vi "Process.vi"(0 "reference in":refnum<class "NI-DAQmx.lvclass">, 5 "error in (no error)":errorcluster) -> (14 "reference out":refnum<class "NI-DAQmx.lvclass">, 19 "error out":errorcluster)   [LabVIEW 2018, in "NI-DAQmx.lvclass"]
uses:
  NI-DAQmx.lvclass
  <vilib>/DAQmx/write.llb/DAQmx Write (Analog 1D DBL 1Chan NSamp).vi
  <vilib>/DAQmx/read.llb/DAQmx Read (Analog 1D Wfm NChan NSamp).vi
  <vilib>/Analysis/5stat.llb/RMS (DBL).vi
  <vilib>/DAQmx/miscellaneous.llb/DAQmx Fill In Error Info.vi
  <vilib>/measure/mascope.llb/Pulse Measurements 1 chan.vi
  <vilib>/measure/mascope.llb/Amplitude and Levels 1 chan.vi
  <resource>/objmgr/daqmx.rc
  <vilib>/measure/NI_MAPro.lvlib
  <vilib>/Analysis/NI_AALPro.lvlib
panel:
  out "Waveform Chart":dbl[][](graph)
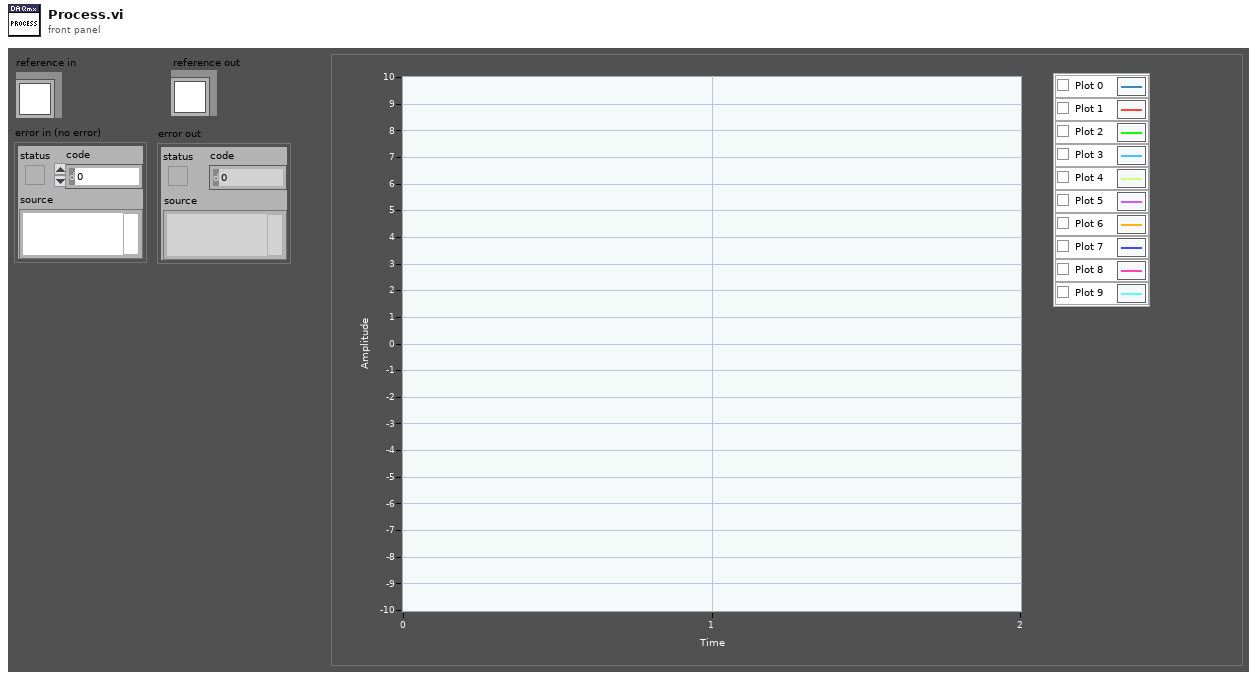
[diagram p1: front panel]
types:
  T1 = cluster{"Event":refnum<event-registration>, "Command":string, "Data":variant}
  T2 = typedef "NI-DAQmx.lvclass/ObjectAttributes.ctl" = cluster{"AI Task":refnum<k21>, "DO Task":refnum<k21>, "AO Task":refnum<k21>, "Latest Values":dbl[], "Signal List":T3[], "PWM Duty Cycle (%)":dbl, "PWM Amplitude (V)":dbl, "PWM Frequency (Hz)":dbl, "DO States":bool[]}
  T3 = typedef "IO Signal List.ctl" = enum16{"Timestamp", "PSU_FB_U_VDC", "PSU_FB_I_AMP", "PSU_FB_W_WATT", "PSU_CMD_U_VDC", "PSU_CMD_I_AMP", "PSU_CMD_OUTPUT", "LCR_PRIMARY", "LCR_SECONDARY", "UV_R_Ohm", "UW_R_Ohm", "VW_R_Ohm", "UV_L_H", "UW_L_H", "VW_L_H", "U_U_VDC", "V_U_VDC", "W_U_VDC", "U_I_AMP", "V_I_AMP", "W_I_AMP", "PWM_CMD_DC_%", "PWM_CMD_VDC", "PWM_CMD_Hz", "PWM_FB_DC_%", "PWM_FB_VDC", "PWM_FB_Hz", "DO_RELAY_U_LCR_A", "DO_RELAY_V_LCR_A", "DO_RELAY_V_LCR_B", "DO_RELAY_W_LCR_B", "DIFF_UV_UW_L_H", "DIFF_UV_VW_L_H", "DIFF_UW_VW_L_H", "DIFF_UV_UW_R_Ohm", "DIFF_UV_VW_R_Ohm", "DIFF_UW_VW_R_Ohm", "DIFF_UV_U_VDC", "DIFF_UW_U_VDC", "DIFF_VW_U_VDC"}
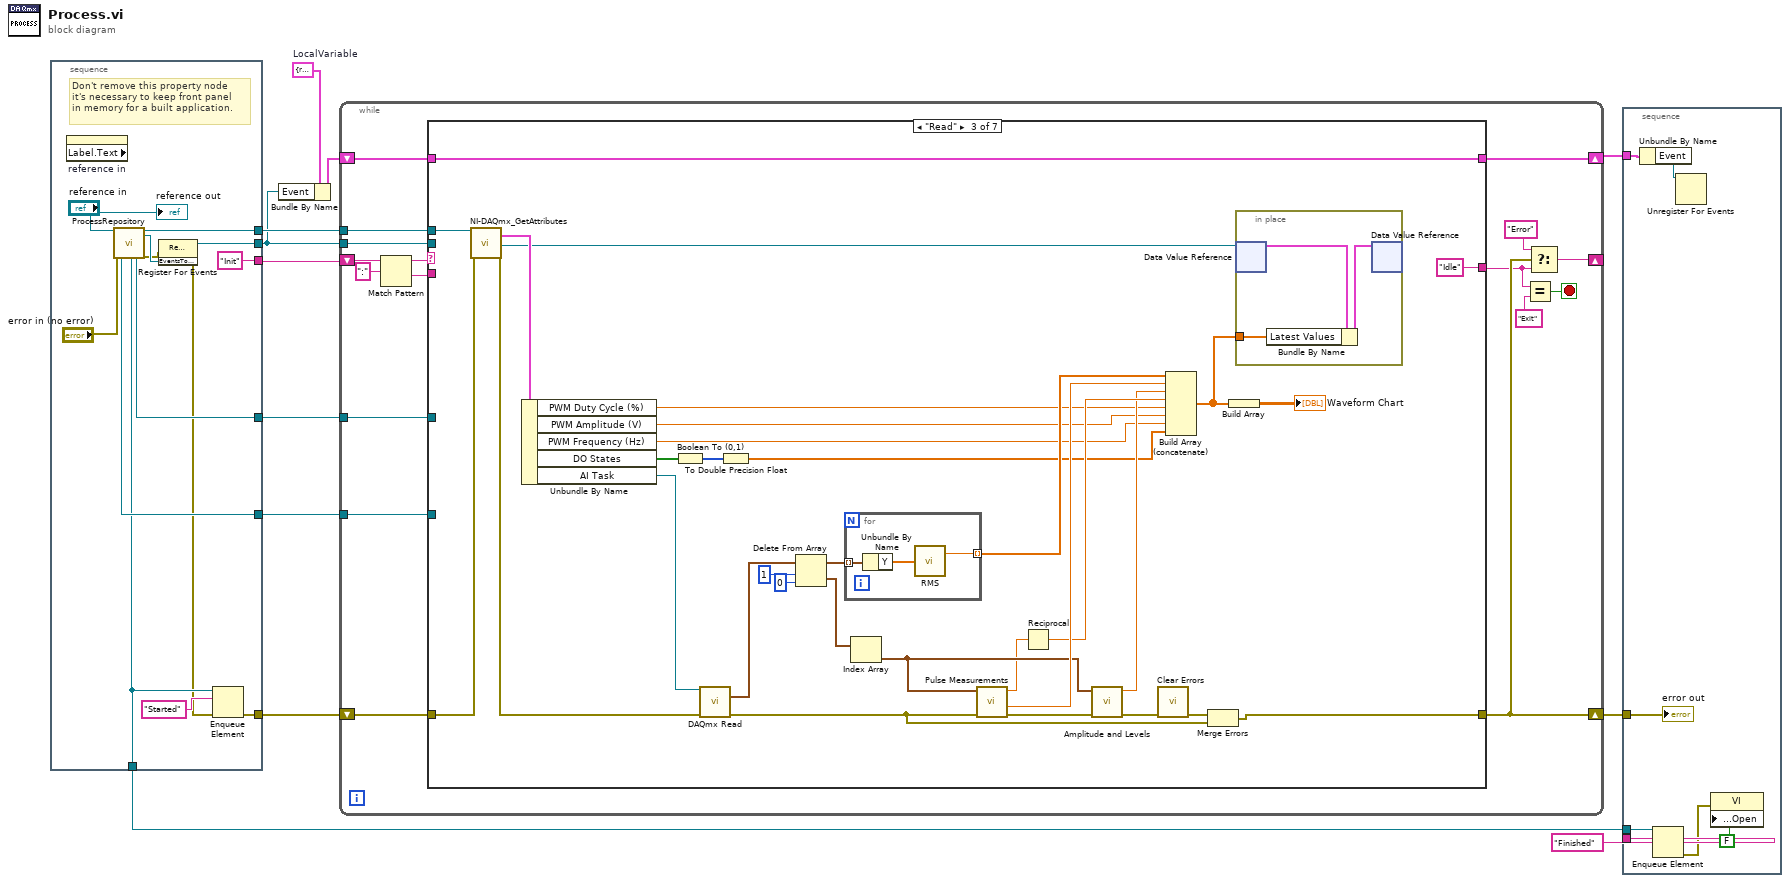
[diagram p0: block diagram]
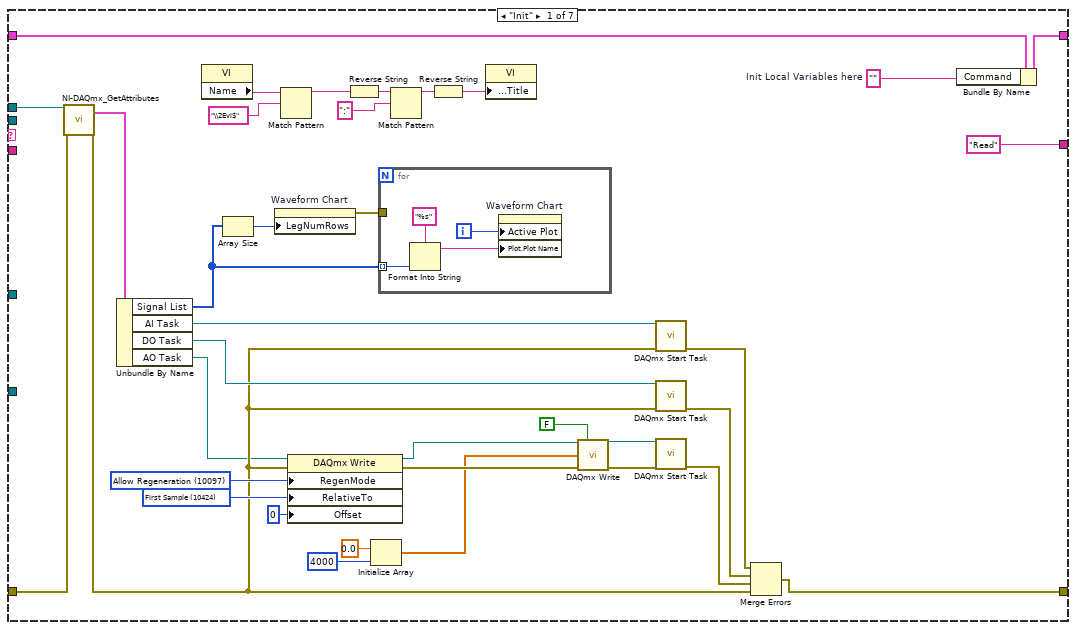
[diagram p2: hidden frame]
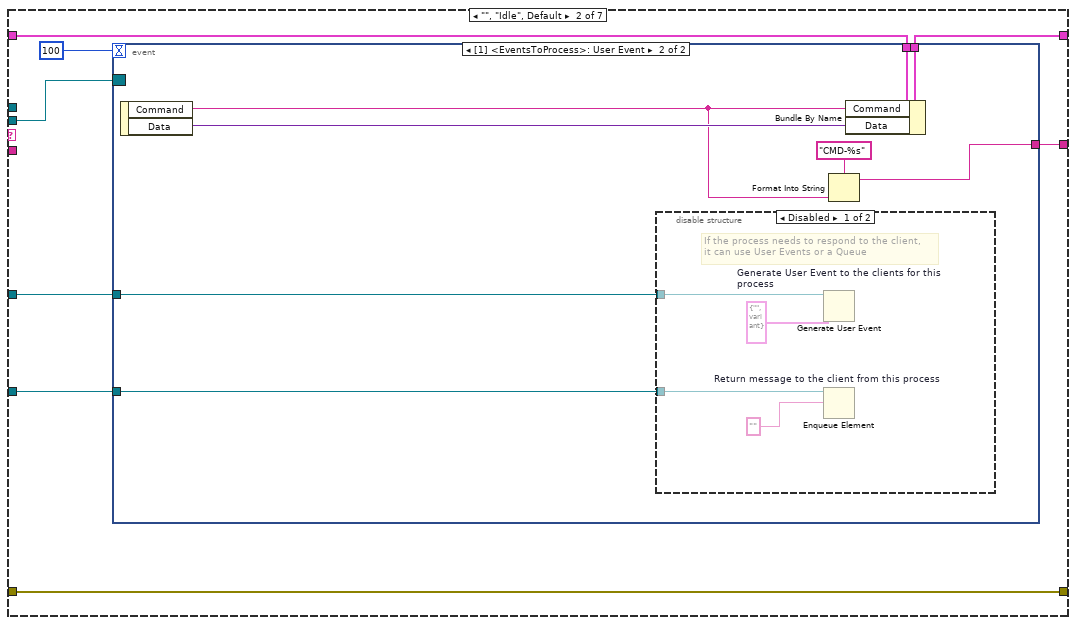
[diagram p3: hidden frame]
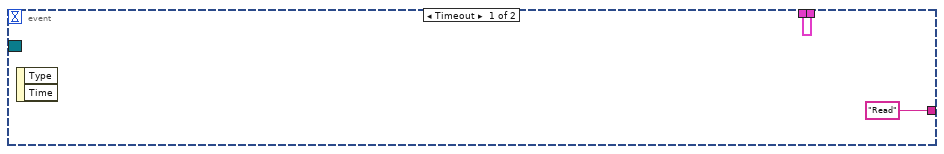
[diagram p4: hidden frame]
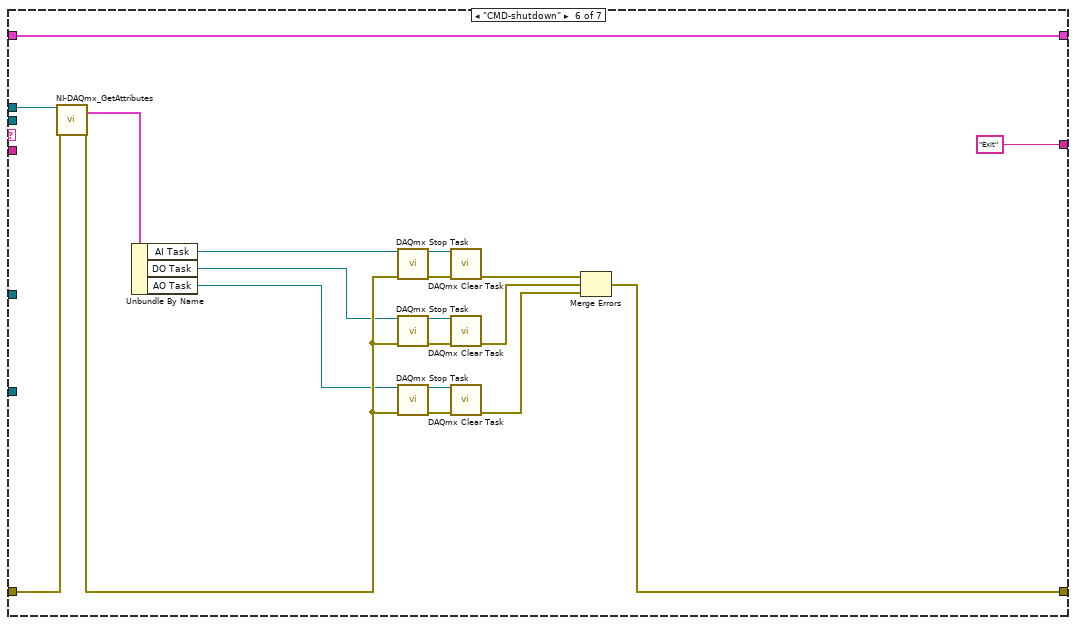
[diagram p8: hidden frame]
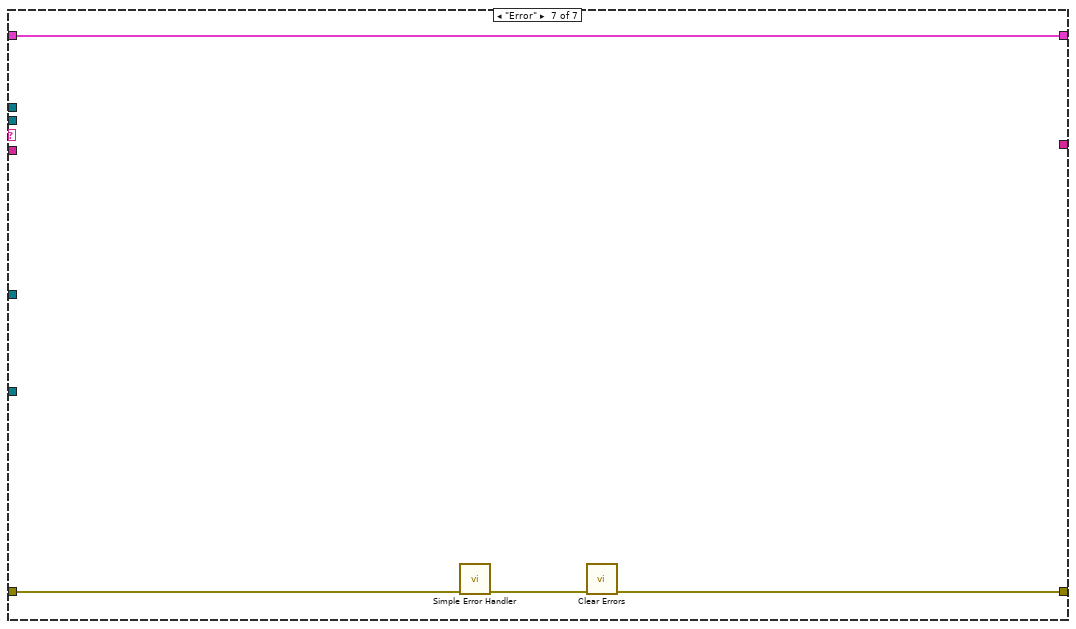
[diagram p9: hidden frame]
diagram:
  w3 = T1 {"Event"=refnum, "Command"="", "Data"=variant}  # LocalVariable
  n1 = stacked-sequence {
    tunnel: [w18] -> w12
    tunnel: [w25] -> w10
    tunnel: [w15] -> w1
    tunnel: [w19] -> w9
    tunnel: ["Init"] -> w8
    tunnel: [w21] -> w6
    tunnel: [w20] -> w5
    frame #0 {
      # "Don't remove this property node\nit's necessary to keep front panel\nin memory for a built application."
      n2 = property on="reference in" class="LVClassControl (strict)" props=["Label", "Text"]() -> ()  [unwired: 2 in, 3 out]
      n3 = call "ProcessRepository.vi"("reference in"="reference in", "error in (no error)"="error in (no error)") -> ("QueueFromProcess"=w20:refnum<queue>, "ProcessSyncQueue"=w19:refnum<queue>, "EventFromProcess"=w21:refnum<user-event>, "reference out"=w25:refnum<class "NI-DAQmx.lvclass">, "EventsToProcess"=w16:refnum<user-event>, "error out"=w14:errorcluster)  [unwired: 10 in, 2 out]
      n4 = register-events(error in=w14, w16) -> (reference out=w15:refnum<event-registration>, error out=w13:errorcluster)  [unwired: 1 in]
      n5 = Enqueue Element(queue=w19, element="Started", error in (no error)=w13) -> (error out=w18:errorcluster)  [unwired: 1 in, 2 out]
      "reference out" <- "reference in"
    }
  }
  n6 = Bundle By Name(cluster=w3, "Event"=w1) -> (w2:T1)
  n7 = while {
    shift-right: [w35] -> w11
    shift-left: w12 -> [w40]
    tunnel: w10 -> [w41]
    tunnel: w1 -> [w42]
    shift-right: [w33] -> _
    shift-left: w8 -> [w38]
    shift-right: [w29] -> w7
    shift-left: w2 -> [w28]
    tunnel: w6 -> [w27]
    tunnel: w5 -> [w26]
    stop <- w30 stop-if-true
    n8 = Match Pattern(string=w38, regular expression=":") -> (before substring=w37:string, after substring=w36:string)  [unwired: 1 in, 2 out]
    n9 = case shown="\"Read\"" w37 {
      tunnel: w40 -> [w67 w86 w133 w144 w146 w160 w168]
      tunnel: [w61 w86 w107 w144 w146 w147 w166] -> w35
      tunnel: w42 -> [_ w83 _ _ _ _ _]
      tunnel: w41 -> [w68 _ w134 _ _ w161 _]
      tunnel: w36 -> [_ _ _ _ _ _ _]
      tunnel: ["Read" ("t") w90 "Idle" ("t") _ _ "Exit" ("y") _] -> w32
      tunnel: [w78 w89 w135 w143 w145 w164 w169] -> w29
      tunnel: w28 -> [w69 w88 w135 w143 w145 w164 w169]
      tunnel: w27 -> [_ w85 _ _ _ _ _]
      tunnel: w26 -> [_ w84 _ _ _ _ _]
      frame "Init" {
        w58 = 10424 items=["First Sample"=10424, "Current Write Position"=10430] ("RelativeTo")
        w59 = 10097 items=["Allow Regeneration"=10097, "Do Not Allow Regeneration"=10158] ("RegenMode")
        w77 = ""  # Init Local Variables here
        n10 = call "NI-DAQmx_GetAttributes.vi"("reference in"=w68, "error in (no error)"=w67) -> ("Data"=w66:T2, "error out"=w56:errorcluster)  [unwired: 14 in, 2 out]
        n11 = Unbundle By Name(w66) -> ("Signal List"=w45:T3[], "AI Task"=w65:refnum<k21>, "DO Task"=w60:refnum<k21>, "AO Task"=w55:refnum<k21>)
        n12 = property class="VI"() -> ("Name"=w76:string)  [unwired: 2 in, 2 out]
        n13 = Array Size(array=w45) -> (size(s)=w44:i32)
        n14 = property on="Waveform Chart" class="WFChart (strict)"("LegNumRows"=w44) -> (error out=w43:errorcluster)  [unwired: 2 in, 1 out]
        n15 = Match Pattern(string=w76, regular expression="\\2Evi$") -> (before substring=w74:string)  [unwired: 1 in, 3 out]
        n16 = property class="DAQmx Write"(reference=w55, error in=w56, "RegenMode"=w59, "RelativeTo"=w58, "Offset"=0) -> (reference out=w52:refnum<k21>, error out=w53:errorcluster)
        n17 = Reverse String(1:w74) -> (0:w73:string)
        n18 = Initialize Array(0.0, 4000 ("samples")) -> (w49:dbl[])
        n19 = for {
          tunnel: w45 -> [w81] mode=indexing
          tunnel: w43 -> [_]
          i -> [w82]
          n20 = Format Into String(format string="%s", w81) -> (resulting string=w79:string)  [unwired: 2 in, 1 out]
          n21 = property on="Waveform Chart" class="WFChart (strict)"("Active Plot"=w82, "Plot.Plot Name"=w79) -> ()  [unwired: 2 in, 2 out]
        }
        n22 = Match Pattern(string=w73, regular expression=":") -> (before substring=w71:string)  [unwired: 1 in, 3 out]
        n23 = Reverse String(1:w71) -> (0:w70:string)
        n24 = property class="VI"("Front Panel.Title"=w70) -> ()  [unwired: 2 in, 2 out]
        n25 = call-poly <vilib>:"DAQmx Write.vi"("task/channels in"=w52, "auto start"=FALSE, "data"=w49, "error in"=w53) -> ("task out"=w47:refnum<k21>, "error out"=w48:errorcluster)  [unwired: 9 in, 1 out]
        n26 = call <vilib>:"DAQmx Start Task.vi"("task/channels in"=w65, "error in"=w56) -> ("error out"=w64:errorcluster)  [unwired: 12 in, 1 out]
        n27 = call <vilib>:"DAQmx Start Task.vi"("task/channels in"=w60, "error in"=w56) -> ("error out"=w63:errorcluster)  [unwired: 12 in, 1 out]
        n28 = call <vilib>:"DAQmx Start Task.vi"("task/channels in"=w47, "error in"=w48) -> ("error out"=w62:errorcluster)  [unwired: 12 in, 1 out]
        n29 = Merge Errors(w64, w63, w62, w56) -> (w61:errorcluster)
        n30 = Bundle By Name(cluster=w69, "Command"=w77) -> (w78:T1)
      }
      frame "", "Idle", Default {
        n31 = event shown="[1] <EventsToProcess>: User Event" {
          selector: w83 -> [_ _]
          dyn-events: _ -> [_ _]
          timeout: 100 -> [_ _]
          tunnel: ["Read" ("t") w96] -> w90
          tunnel: w88 -> [w91 w100]
          tunnel: [w91 w99] -> w89
          tunnel: w85 -> [_ w94]
          tunnel: w84 -> [_ w93]
          event Timeout {
            n32 = event-data() -> ()  [unwired: 1 in, 2 out]
          }
          event User Event {
            n33 = event-data() -> ("Command"=w95:string, "Data"=w98:variant)  [unwired: 1 in]
            n34 = disable-structure shown="Disabled" {
              disable-tunnel: w94 -> [w104 _]
              disable-tunnel: w93 -> [w103 _]
              frame Disabled {
                # "If the process needs to respond to the client,\nit can use User Events or a Queue"
                n35 = Generate User Event "Generate User Event to the clients for this process"(user event=w104, event data cluster=cluster{"Command":string, "Data":variant} {"Command"="", "Data"=variant} ("event data")) -> ()  [unwired: 2 in, 2 out]
                n36 = Enqueue Element "Return message to the client from this process"(queue=w103, element="") -> ()  [unwired: 2 in, 3 out]
              }
              frame Enabled {
              }
            }
            n37 = Format Into String(format string="CMD-%s", w95) -> (resulting string=w96:string)  [unwired: 2 in, 1 out]
            n38 = Bundle By Name(cluster=w100, "Command"=w95, "Data"=w98) -> (w99:T1)
          }
        }
      }
      frame "Read" {
        n39 = call "NI-DAQmx_GetAttributes.vi"("reference in"=w134, "error in (no error)"=w133) -> ("Data"=w132:T2, "DataRef"=w130:refnum<data-value>, "error out"=w131:errorcluster)  [unwired: 14 in, 1 out]
        n40 = Unbundle By Name(w132) -> ("PWM Duty Cycle (%)"=w117:dbl, "PWM Amplitude (V)"=w116:dbl, "PWM Frequency (Hz)"=w111:dbl, "DO States"=w114:bool[], "AI Task"=w115:refnum<k21>)
        n41 = Boolean To (0,1)(Boolean=w114) -> (0, 1=w113:i16[])
        n42 = call-poly <vilib>:"DAQmx Read.vi"("task/channels in"=w115, "error in"=w131) -> ("data"=w125:waveform(dbl)[], "error out"=w109:errorcluster)  [unwired: 11 in, 1 out]
        n43 = To Double Precision Float(number=w113) -> (double precision float=w112:dbl[])
        n44 = Delete From Array(array=w125, length=1, index=0) -> (deleted portion=w123:waveform(dbl)[], array with subset deleted=w124:waveform(dbl)[])
        n45 = for {
          tunnel: w124 -> [w139] mode=indexing
          tunnel: [w137] -> w129 mode=indexing
          n46 = Unbundle By Name(w139) -> ("Y"=w138:dbl[])
          n47 = call-poly <vilib>:"RMS.vi"("X"=w138) -> ("rms value"=w137:dbl)  [unwired: 1 out]
        }
        n48 = Index Array(array=w123) -> (element=w122:waveform(dbl))  [unwired: 1 in]
        n49 = call-poly <vilib>:"Pulse Measurements.vi"("error in (no error)"=w109, "signal in"=w122) -> ("error out"=w121:errorcluster, "duty cycle"=w128:dbl, "period"=w120:dbl)  [unwired: 5 in, 2 out]
        n50 = Reciprocal(x=w120) -> (1/x=w119:dbl)
        n51 = call-poly <vilib>:"Amplitude and Levels.vi"("error in (no error)"=w121, "signal in"=w122) -> ("error out"=w110:errorcluster, "amplitude"=w118:dbl)  [unwired: 6 in, 2 out]
        n52 = call <vilib>:"Clear Errors.vi"("error in (no error)"=w110) -> ("error out"=w108:errorcluster)  [unwired: 5 in, 1 out]
        n53 = Build Array (concatenate)(w129, w128, w118, w119, w117, w116, w111, w112) -> (w106:dbl[])
        n54 = Merge Errors(w108, w109) -> (w107:errorcluster)
        n55 = Build Array(w106) -> (→"Waveform Chart":dbl[][])
        n56 = in-place {
          in-place-border: w106 -> [w140]
          n57 = in-place-dvr #1(w130) -> (w142:T2)  [unwired: 1 out]
          n58 = Bundle By Name(cluster=w142, "Latest Values"=w140) -> (w141:T2)
          n59 = in-place-dvr #1(w141) -> ()  [unwired: 2 out]
        }
      }
      frame "---- COMMANDS START----" {
      }
      frame "----- COMMANDS END ----" {
      }
      frame "CMD-shutdown" {
        n60 = call "NI-DAQmx_GetAttributes.vi"("reference in"=w161, "error in (no error)"=w160) -> ("Data"=w162:T2, "error out"=w154:errorcluster)  [unwired: 14 in, 2 out]
        n61 = Unbundle By Name(w162) -> ("AI Task"=w159:refnum<k21>, "DO Task"=w152:refnum<k21>, "AO Task"=w151:refnum<k21>)
        n62 = call <vilib>:"DAQmx Stop Task.vi"("task/channels in"=w159, "error in"=w154) -> ("task out"=w163:refnum<k21>, "error out"=w153:errorcluster)  [unwired: 12 in]
        n63 = call <vilib>:"DAQmx Stop Task.vi"("task/channels in"=w152, "error in"=w154) -> ("task out"=w158:refnum<k21>, "error out"=w155:errorcluster)  [unwired: 12 in]
        n64 = call <vilib>:"DAQmx Stop Task.vi"("task/channels in"=w151, "error in"=w154) -> ("task out"=w157:refnum<k21>, "error out"=w156:errorcluster)  [unwired: 12 in]
        n65 = call <vilib>:"DAQmx Clear Task.vi"("task in"=w163, "error in"=w153) -> ("error out"=w150:errorcluster)  [unwired: 13 in]
        n66 = call <vilib>:"DAQmx Clear Task.vi"("task in"=w158, "error in"=w155) -> ("error out"=w149:errorcluster)  [unwired: 13 in]
        n67 = call <vilib>:"DAQmx Clear Task.vi"("task in"=w157, "error in"=w156) -> ("error out"=w148:errorcluster)  [unwired: 13 in]
        n68 = Merge Errors(w150, w149, w148) -> (w147:errorcluster)
      }
      frame "Error" {
        n69 = call <vilib>:"Simple Error Handler.vi"("error in (no error)"=w168) -> ("error out"=w167:errorcluster)  [unwired: 4 in, 4 out]
        n70 = call <vilib>:"Clear Errors.vi"("error in (no error)"=w167) -> ("error out"=w166:errorcluster)  [unwired: 5 in, 1 out]
      }
    }
    n71 = Equal?(x=w32, y="Exit") -> (x = y?=w30:bool)
    n72 = Select(t="Error", s=w35, f=w32) -> (s? t:f=w33:string)
  }
  n73 = stacked-sequence {
    tunnel: w11 -> [w176]
    tunnel: w9 -> [w172]
    tunnel: w7 -> [w175]
    tunnel: "Finished" ("element") -> [w170]
    frame #0 {
      n74 = Unbundle By Name(w175) -> ("Event"=w174:refnum<event-registration>)
      n75 = Enqueue Element(queue=w172, element=w170) -> (error out=w171:errorcluster)  [unwired: 2 in, 2 out]
      n76 = Unregister For Events(event registration refnum=w174) -> ()  [unwired: 1 in, 1 out]
      n77 = property class="VI"(error in=w171, "Front Panel.Open"=FALSE ("Front Panel Window:Open")) -> ()  [unwired: 1 in, 2 out]
      "error out" <- w176
    }
  }
